vi "PI STAGE TEST.vi"() -> ()   [LabVIEW 2018]
panel:
  out "Error Description":string
  out "READY AXES":string[](array[string])
  out "4L":bool
  out "3L":bool
  out "2L":bool
  out "1L":bool
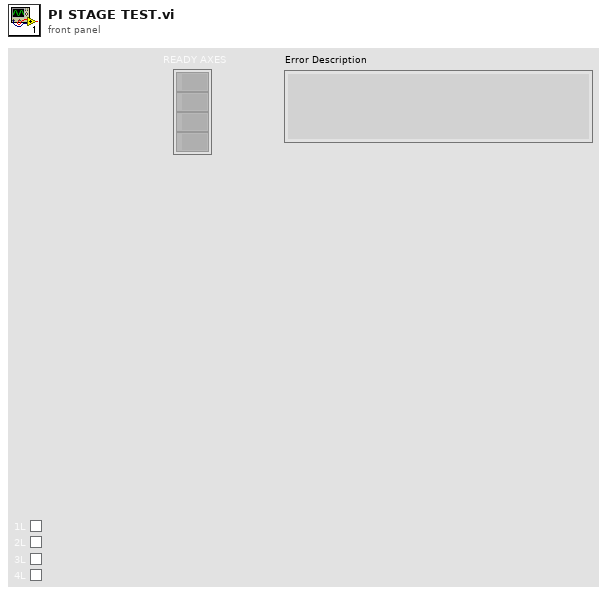
[diagram p1: front panel]
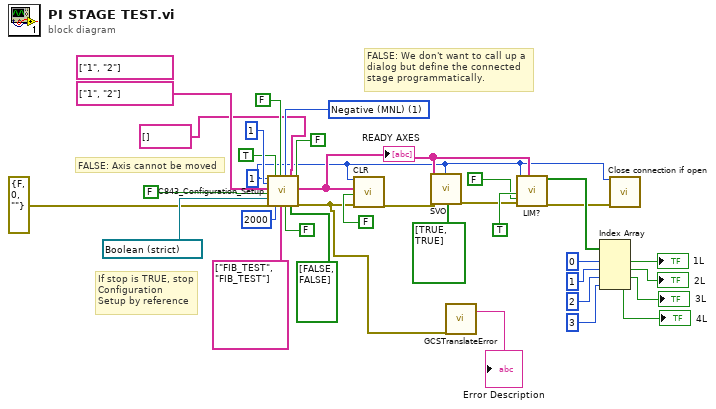
[diagram p0: block diagram]
diagram:
  w3 = 1 ("System no.")
  (unwired) string[] ["1", "2"]
  w31 = u16 1 items=["Positive (MPL)", "Negative (MNL)"] ("Limit switch selection")
  # "If stop is TRUE, stop \nConfiguration\nSetup by reference"
  # "FALSE: We don't want to call up a \ndialog but define the connected\nstage programmatically."
  # "FALSE: Axis cannot be moved"
  n1 = call "C843_Configuration_Setup.vi"("System no."=w3, "C-843 Board No."=1, "Axes to move"=string[] ["1", "2"], "All axes?"=FALSE, "Stop refnum"=refnum<vi> refnum, "error in"=errorcluster {"status"=FALSE, "code"=0, "source"=""}, "C-843 version"=TRUE, "Timeout"=u32 2000, "Use dialog to define\nconnected stages?"=FALSE ("Use dialog to define\nconnected stages?"), "Stage names input"=string[] ["FIB_TEST", "FIB_TEST"], "Limit switch selection"=w31, "Define home?"=FALSE, "RON Affected axes"=string[] [], "Reference mode"=bool[] [FALSE, FALSE], "Move to middle?"=FALSE) -> ("Conn. \nAxes"=w7:string[], "error out"=w2:errorcluster)  [unwired: 3 out]
  "READY AXES" <- w7
  n2 = call "CLR.vi"("System no."=w3, "CLR axes"=w7, "All axes?"=FALSE, "error in"=w2) -> ("error out"=w6:errorcluster)  [unwired: 1 in, 14 out]
  n3 = call "SVO.vi"("System no."=w3, "Axes to command"=w7, "Servo mode"=bool[] [TRUE, TRUE], "error in"=w6) -> ("error out"=w17:errorcluster)  [unwired: 1 in, 14 out]
  n4 = call "GCSTranslateError.vi"("error in"=w2) -> ("Error Description"=→"Error Description":string)  [unwired: 16 in, 2 out]
  n5 = call "LIM?.vi"("System no."=w3, "Axes to query"=w7, "All axes?"=TRUE, "Axis identifier?"=FALSE, "error in"=w17) -> ("Axis with limit switch?"=w29:bool[], "error out"=w4:errorcluster)  [unwired: 13 out]
  n6 = Index Array(array=w29, index #1=0 ("index"), index #2=1 ("index"), index #3=2 ("index"), index #4=3 ("index")) -> (element #1=→"1L":bool, element #2=→"2L":bool, element #3=→"3L":bool, element #4=→"4L":bool)
  n7 = call "Close connection if open.vi"("System no."=w3, "error in"=w4) -> ()  [unwired: 1 in, 17 out]
